vi "Focus Initialize.vi"(8 "error in (no error)":errorcluster, 10 "Motion Settings":T1, 11 "ArduinoFocus in":refnum<class "ArduinoFocus.lvclass">) -> (0 "error out":errorcluster, 1 "Motor Positions":i32[](array[numeric]), 2 "Device Name":string, 3 "ArduinoFocus out":refnum<class "ArduinoFocus.lvclass">)   [LabVIEW 2022 SP3, in "ArduinoFocus.lvclass"]
uses:
  ArduinoFocus.lvclass
  Focus cluster Motion Settings.ctl
  Arduino Focus cluster Settings.ctl
  Motor Control Driver/arduino Motor Control cluster Command.ctl
  ArduinoFocus.lvclass/ArduinoFocus.ctl
  Focus Class/Focus Class.lvclass
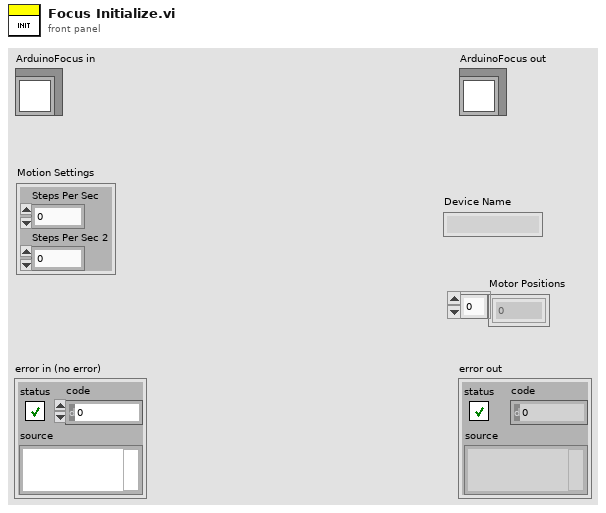
[diagram p1: front panel]
types:
  T1 = typedef "Focus cluster Motion Settings.ctl" = cluster{"Steps Per Sec":i32, "Steps Per Sec 2":i32}
  T2 = typedef "ArduinoFocus.lvclass/Arduino Focus cluster Settings.ctl" = cluster{"Port":refnum<visa-resource-name>, "Homing Parameters":T3, "Positions":i32[], "Homed":bool[]}
  T3 = typedef "arduino Motor Control cluster Command.ctl" = cluster{"Direction":bool, "NUMBER OF  STEPS":u32, "SPEED STEPS/SEC":u16, "ACC/DECEL STEPS/SEC^2":u16, "EN/DIS?":bool}
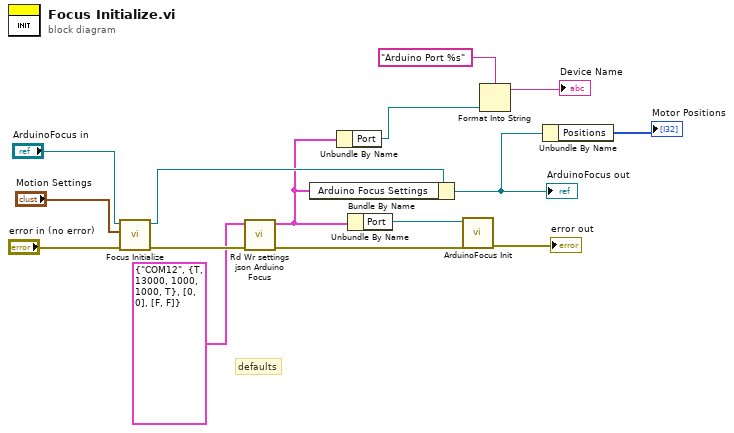
[diagram p0: block diagram]
diagram:
  # "defaults"
  n1 = call-parent "Focus Initialize.vi"("error in (no error)"="error in (no error)", "Motion Settings"="Motion Settings", "Focus Class in"="ArduinoFocus in") -> ("error out"=w9:errorcluster, "Focus Class out"=w12:refnum<class "ArduinoFocus.lvclass">)  [unwired: 5 in, 2 out]
  n2 = call "Rd Wr settings json Arduino Focus.vi"("error in (no error)"=w9, "Arduino Focus Settings"=T2 {"Port"="COM12", "Homing Parameters"={"Direction"=TRUE, "NUMBER OF  STEPS"=13000, "SPEED STEPS/SEC"=1000, "ACC/DECEL STEPS/SEC^2"=1000, "EN/DIS?"=TRUE}, "Positions"=[0, 0], "Homed"=[FALSE, FALSE]}) -> ("error out"=w8:errorcluster, "Arduino Focus Settings"=w3:T2)  [unwired: 8 in]
  n3 = Bundle By Name(cluster=w12, "Arduino Focus Settings"=w3) -> (w6:refnum<class "ArduinoFocus.lvclass">)
  "ArduinoFocus out" <- w6
  n4 = Unbundle By Name(w3) -> ("Port"=w2:refnum<visa-resource-name>)
  n5 = Unbundle By Name(w3) -> ("Port"=w11:refnum<visa-resource-name>)
  n6 = call "ArduinoFocus Init.vi"("error in (no error)"=w8, "VISA resource name"=w11) -> ("value out"=→"error out":errorcluster)  [unwired: 8 in, 1 out]
  n7 = Format Into String(format string="Arduino Port %s", w2) -> (resulting string=→"Device Name":string)  [unwired: 2 in, 1 out]
  n8 = Unbundle By Name(w6) -> ("Positions"=→"Motor Positions":i32[])
